vi "WFT PS Set Voltage.vi"(8 "Error In":errorcluster, 10 "Voltage":dbl=3.3 format="%#_13g", 11 "WaveForms Session In":T1) -> (0 "Error Out":errorcluster, 3 "WaveForms Session Out":T1)   [LabVIEW 2020, in "lv_waveforms_toolkit.lvlib"]
uses:
  lv_waveforms_toolkit.lvlib
  WFT Session.ctl
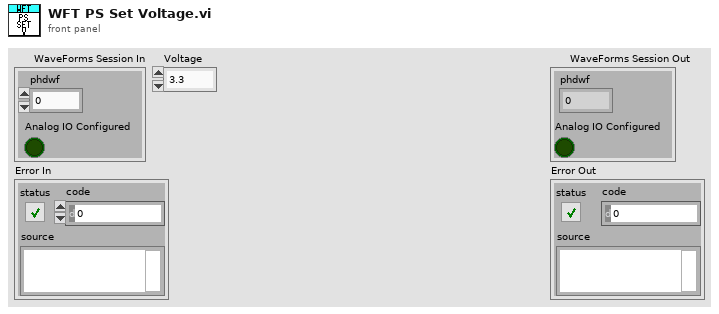
[diagram p1: front panel]
types:
  T1 = typedef "lv_waveforms_toolkit.lvlib/WFT Session.ctl" = cluster{"phdwf":i32, "Analog IO Configured":bool}
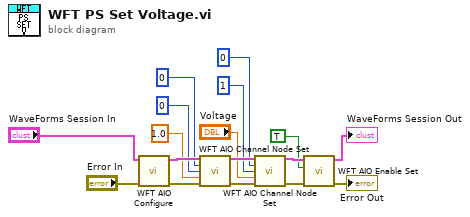
[diagram p0: block diagram]
diagram:
  n1 = call "WFT AIO Configure.vi"("Error In"="Error In", "WaveForms Session In"="WaveForms Session In") -> ("Error Out"=w11:errorcluster, "WaveForms Session Out"=w17:T1)  [unwired: 7 in, 1 out]
  n2 = call "WFT AIO Channel Node Set.vi"("WaveForms Session In"=w17, "idxChannel"=0, "idxNode"=0, "value"=1.0, "Error In"=w11) -> ("WaveForms Session Out"=w16:T1, "Error Out"=w12:errorcluster)  [unwired: 8 in, 1 out]
  n3 = call "WFT AIO Channel Node Set.vi"("WaveForms Session In"=w16, "idxChannel"=0, "idxNode"=1, "value"="Voltage", "Error In"=w12) -> ("WaveForms Session Out"=w15:T1, "Error Out"=w13:errorcluster)  [unwired: 8 in, 1 out]
  n4 = call "WFT AIO Enable Set.vi"("Error In"=w13, "fMasterEnable"=TRUE, "WaveForms Session In"=w15) -> ("Error Out"=→"Error Out":errorcluster, "WaveForms Session Out"=→"WaveForms Session Out":T1)  [unwired: 6 in, 1 out]
